vi "flattenForceToXML.vi"   [LabVIEW 2012, in "UnitsAndXML.lvlib"]
doc: "Generates an XML string for <B>force</B> in the unit specified in <B>forceUnitInXML</B>. Connect <B>force</B> and <B>forceAgain</B> to the same source. The VI uses <B>forceAgain</B> to obtain the data name."
uses:
  <userlib>/Common/UnitsAndXML/UnitsAndXML.lvlib
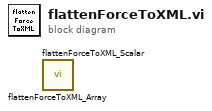
[diagram p0: block diagram]
diagram:
  n1 = call <userlib>:"flattenForceToXML_Array.vi"() -> ()  [unwired: 10 in, 2 out]
  n2 = call <userlib>:"flattenForceToXML_Scalar.vi"() -> ()  [unwired: 10 in, 2 out]
